vi "Send Message, String Payload.vi"(0 "IPEndPoint":T1, 7 "Message":string, 9 "Payload":string="{}", 11 "error in (no error)":errorcluster) -> (4 "IPEndPoint thru":T1, 15 "error out":errorcluster)   [LabVIEW 2020, in "epl-network.lvlib"]
uses:
  epl-network.lvlib
  Typedefs/IPEndPoint.ctl
  Typedefs/TCP Message.ctl
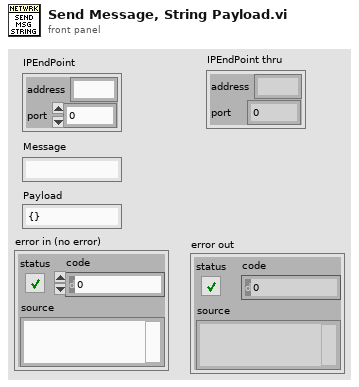
[diagram p1: front panel]
types:
  T1 = typedef "epl-network.lvlib/IPEndPoint.ctl" = cluster{"address":string, "port":i32}
  T2 = typedef "epl-network.lvlib/TCP Message.ctl" = cluster{"Code":i32, "Command":string, "Payload":string}
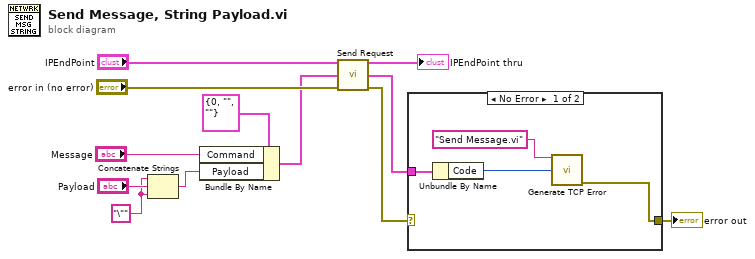
[diagram p0: block diagram]
diagram:
  w2 = "\""
  n1 = Concatenate Strings(w2, "Payload", w2) -> (w1:string)
  n2 = Bundle By Name(cluster=T2 {"Code"=0, "Command"="", "Payload"=""} ("TCPMessage"), "Command"="Message", "Payload"=w1) -> (w8:T2)
  n3 = call "Send Request.vi"("IPEndPoint"="IPEndPoint", "TCPMessage"=w8, "error in (no error)"="error in (no error)") -> ("IPEndPoint thru"=→"IPEndPoint thru":T1, "Response"=w5:T2, "error out"=w6:errorcluster)  [unwired: 10 in]
  n4 = case shown="No Error" w6 {
    selector: w6 -> [_ w17]
    tunnel: w5 -> [w16 _]
    tunnel: [w14 w17] -> w4
    frame No Error {
      n5 = Unbundle By Name(w16) -> ("Code"=w15:i32)
      n6 = call "Generate TCP Error.vi"("VI Name"="Send Message.vi", "TCP response code"=w15) -> ("error out"=w14:errorcluster)  [unwired: 13 in]
    }
    frame Error {
    }
  }
  "error out" <- w4
